vi "NI VeriStand - Get Item Parent.vi"(8 "error in (no error)":errorcluster, 11 "Item Ref in":T1 format="%.0x") -> (0 "error out":errorcluster, 2 "Parent Ref":T1 format="%.0x", 3 "Item Ref out":T1 format="%.0x", 4 "Found":bool)   [LabVIEW 2020, in "Custom Device Offline API.lvlib"]
uses:
  <vilib>/NI VeriStand/Custom Device Offline API/Custom Device Offline API.lvlib
  <vilib>/NI VeriStand/Custom Device API/Custom Device Item Ref.ctl
  NationalInstruments.VeriStand.SystemDefinitionAPI
  <vilib>/NI VeriStand/Custom Device API/Custom Device API.lvlib
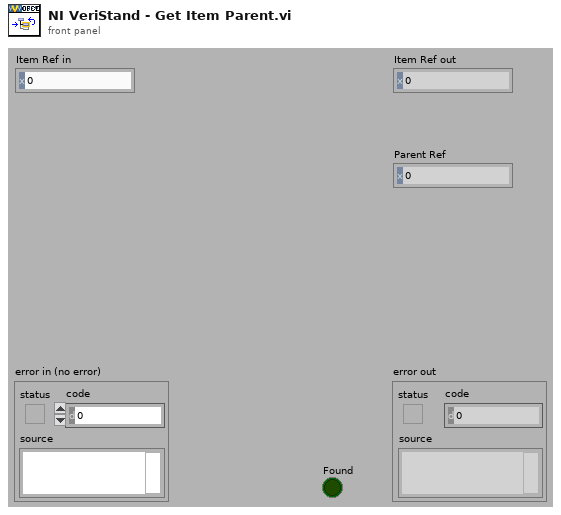
[diagram p1: front panel]
types:
  T1 = typedef "Custom Device API.lvlib/Custom Device Item Ref.ctl" = u64
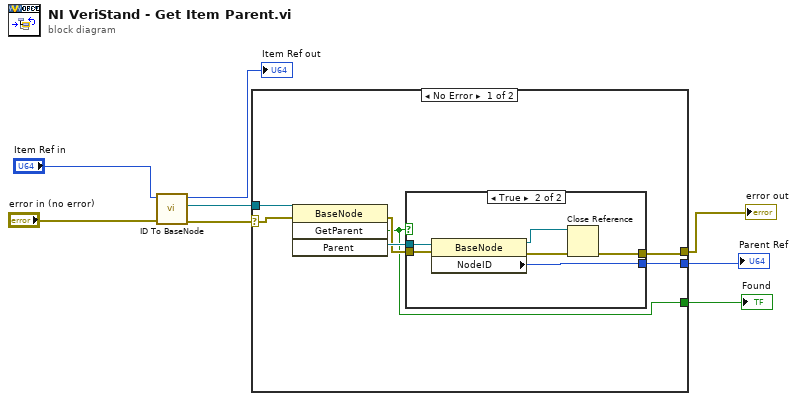
[diagram p0: block diagram]
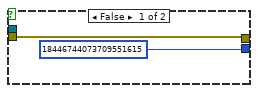
[diagram p2: hidden frame]
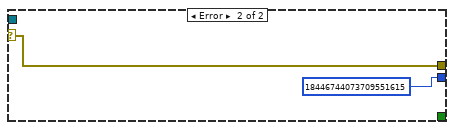
[diagram p3: hidden frame]
diagram:
  n1 = call <vilib>:"ID To BaseNode.vi"("error in (no error)"="error in (no error)", "ID in"="Item Ref in") -> ("error out"=w6:errorcluster, "BaseNode"=w4:refnum<k24>, "ID out"=→"Item Ref out":u64)  [unwired: 7 in]
  n2 = case shown="No Error" w6 {
    selector: w6 -> [w14 w25]
    tunnel: w4 -> [w15 _]
    tunnel: [w11 T1 18446744073709551615 ("Parent Ref")] -> w1
    tunnel: [w10 w25] -> w3
    tunnel: [w9 _] -> w2
    frame No Error {
      n3 = invoke class="BaseNode" method="GetParent"(reference=w15, error in=w14) -> (error out=w12:errorcluster, "GetParent"=w9:bool, "Parent"=w13:refnum<k24>)  [unwired: 2 in, 1 out]
      n4 = case shown="True" w9 {
        tunnel: w13 -> [_ w23]
        tunnel: w12 -> [w17 w22]
        tunnel: [T1 18446744073709551615 ("Parent Ref") w21] -> w11
        tunnel: [w17 w18] -> w10
        frame False {
        }
        frame True {
          n5 = property class="BaseNode"(reference=w23, error in=w22) -> (reference out=w20:refnum<k24>, error out=w19:errorcluster, "NodeID"=w21:u64)
          n6 = Close Reference(reference=w20, error in (no error)=w19) -> (error out=w18:errorcluster)
        }
      }
    }
    frame Error {
    }
  }
  "error out" <- w3
  "Found" <- w2
  "Parent Ref" <- w1
